vi "test-kalman-filter.vi"() -> (3 "ALL TESTS PASSED":bool)   [LabVIEW 2019]
uses:
  <vilib>/Rock Robotics/WPI/ThirdParty/JAS_Junk/TrajLib/LINEAR_SYSTEM.ctl
  <vilib>/Analysis/Matrix/Datatypes/RealMatrix.ctl
  <vilib>/Rock Robotics/WPI/ThirdParty/JAS_Junk/TrajLib/KALMAN_FILTER.ctl
  <vilib>/Rock Robotics/WPI/ThirdParty/JAS_Junk/TrajLib/Rotation_CreateAngle.vi
  <vilib>/Rock Robotics/WPI/ThirdParty/JAS_Junk/TrajLib/Translation_Create.vi
  <vilib>/Rock Robotics/WPI/ThirdParty/JAS_Junk/TrajLib/MatrixHelper_CoerceSize.vi
  <vilib>/Analysis/1siggen.llb/Gaussian White Noise.vi
  <vilib>/Analysis/Matrix/Numeric/Subtract/Subtract - RM,RM.vi
  <vilib>/Analysis/Matrix/Numeric/Add/Add - RM,RM.vi
  <vilib>/Rock Robotics/WPI/ThirdParty/JAS_Junk/TrajLib/Trajectory_Library.lvlib
  <vilib>/Analysis/Matrix/NI_Matrix.lvlib
panel:
  out "WhiteNoise":T1
  out "Error 3C":bool
  out "KalFilt Error 3B":bool
  out "KalFilt Error 3A":bool
  out "Test 1 Passed":bool
  out "max value 4B":dbl
  out "max value 4A":dbl
  out "Test 4 Passed":bool
  out "xHat 4":cluster{dbl[], dbl[]}(graph)
  out "Measurements 4":cluster{dbl[], dbl[]}(graph)
  out "Error 4A":bool
  out "Error 4B":bool
  out "KalFilt Error 4":bool
  out "KalFilt Test 4":T2
  out "max value 3B":dbl
  out "max value 3A":dbl
  out "Test 3 Passed":bool
  out "xHats 3":cluster{dbl[], dbl[]}(graph)
  out "Measurements 3":cluster{dbl[], dbl[]}(graph)
  out "Error 3A":bool
  out "Error 3B":bool
  out "KalFilt Error 3":bool
  out "KalFilt Test 3":T2
  out "Test 2 Passed":bool
  out "xHat 2":cluster{dbl[], dbl[]}(graph)
  out "Measurements 2":cluster{dbl[], dbl[]}(graph)
  out "Error 2B":bool
  out "Error 2A":bool
  out "KalFilt Error 2":bool
  out "KalFilt Test 2":T2
  out "KalFilt Error 1":bool
  out "KalFilt Test1":T2
  out "SwervObservError":bool
  out "SwervObservSystem":T3
  out "EllevError":bool
  out "ElevatorSystem":T3
  # "KALMAN FILTER"
  # "Steady State Gain  \n<States,Outputs>"
  # "State Estimate <Statess,1>"
  # "<States,States>"
  # "<States,Inputs>"
  # "<Outputs,States>"
  # "<Outputs,Inputs>"
  # "Steady State Gain  \n<States,Outputs>"
  # "State Estimate <Statess,1>"
  # "<States,States>"
  # "<States,Inputs>"
  # "<Outputs,States>"
  # "<Outputs,Inputs>"
  # "Steady State Gain  \n<States,Outputs>"
  # "State Estimate <Statess,1>"
  # "<States,States>"
  # "<States,Inputs>"
  # "<Outputs,States>"
  # "<Outputs,Inputs>"
  # "Steady State Gain  \n<States,Outputs>"
  # "State Estimate <Statess,1>"
  # "<States,States>"
  # "<States,Inputs>"
  # "<Outputs,States>"
  # "<Outputs,Inputs>"
  # "<States,States>"
  # "<States,Inputs>"
  # "<Outputs,States>"
  # "<Outputs,Inputs>"
  # "<States,States>"
  # "<States,Inputs>"
  # "<Outputs,States>"
  # "<Outputs,Inputs>"
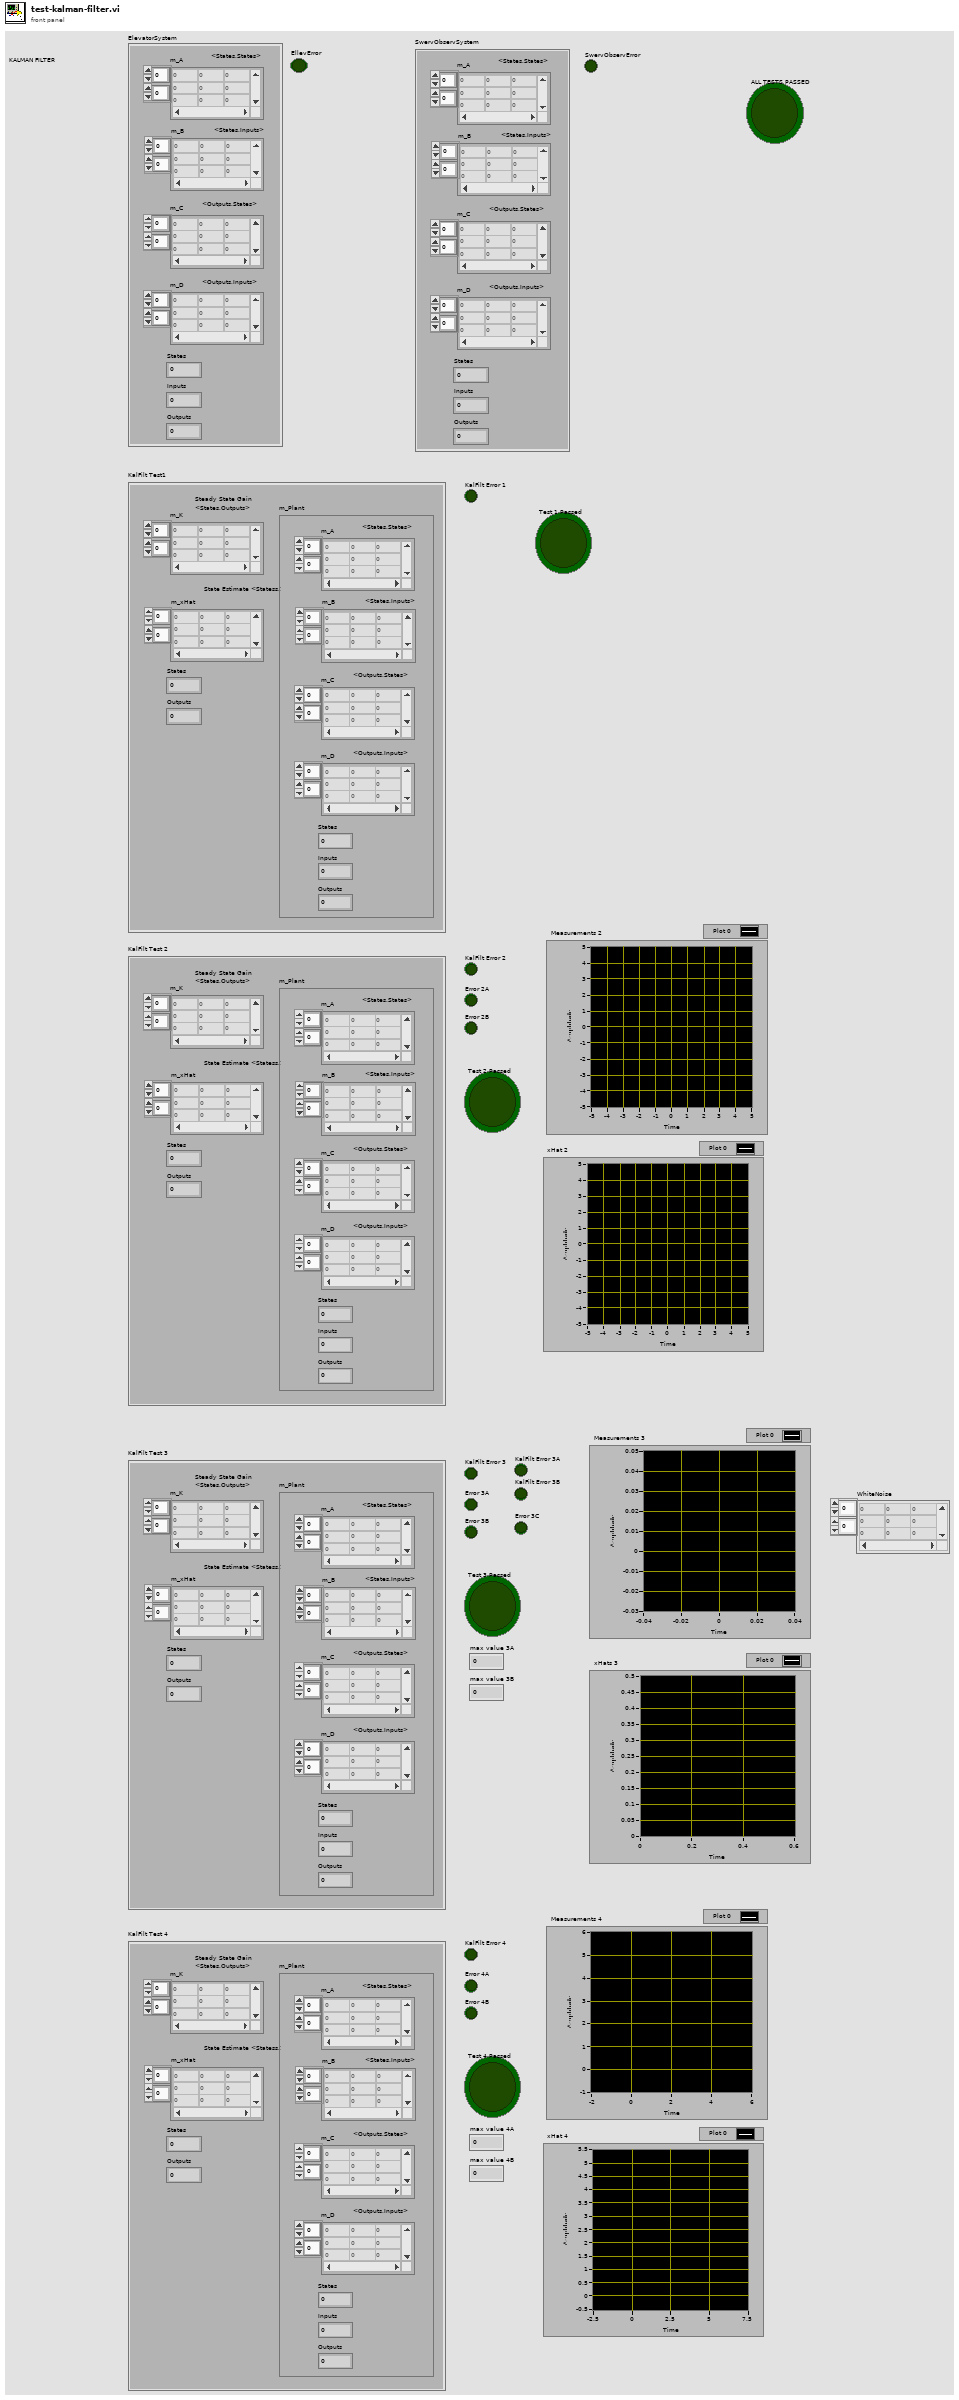
[diagram p1: front panel]
types:
  T1 = typedef "NI_Matrix.lvlib/RealMatrix.ctl" = dbl[][]
  T2 = typedef "Trajectory_Library.lvlib/KALMAN_FILTER.ctl" = cluster{"m_K":T1, "m_xHat":T1, "States":i32, "Outputs":i32, "m_Plant":T3}
  T3 = typedef "Trajectory_Library.lvlib/LINEAR_SYSTEM.ctl" = cluster{"m_A":T1, "m_B":T1, "m_C":T1, "m_D":T1, "States":i32, "Inputs":i32, "Outputs":i32}
  T4 = typedef "Trajectory_Library.lvlib/TRAJ_CONFIG.ctl" = cluster{"MaxVelocity":dbl, "Max Acceleration":dbl, "StartVelocity":dbl, "End Velocity":dbl, "Reversed":bool, "DiffDrKineConstntDefined":bool, "CentAcellConstntDefined":bool, "DiffDrVoltConstntDefined":bool, "DIFF_DRIVE_KINE_CONSTRAINT":T5, "CENTRIPETAL_ACCEL_CONSTRAINT":T7, "SwerveDrKineConstntDefined":bool, "SWERVE_DRIVE_KINE_CONSTRAINT":T8, "DIFF_DRIVE_VOLTAGE_CONSTRAINT":T11, "MECANUM_DRIVE_KINE_CONSTRAINT":T13, "MecanumDrKineConstntDefined":bool}
  T5 = typedef "Trajectory_Library.lvlib/TRAJ_CONSTRAINT_DIIF_DRIVE_KINEMATICS.ctl" = cluster{"Max Speed (M/S)":dbl, "DIFF_DRIVE_KINEMATICS":T6}
  T6 = typedef "Trajectory_Library.lvlib/DIFF_DRIVE_KINEMATICS.ctl" = cluster{"TrackWidth_Meters":dbl}
  T7 = typedef "Trajectory_Library.lvlib/TRAJ_CONSTRAINT_CENTRIPETAL_ACCEL.ctl" = cluster{"Max Cent Accel":dbl}
  T8 = typedef "Trajectory_Library.lvlib/TRAJ_CONSTRAINT_SWERVE_DRIVE_KINEMATICS.ctl" = cluster{"Max Speed (M/S)":dbl, "SwerveKinematics":T9}
  T9 = typedef "Trajectory_Library.lvlib/SWERVE_DRIVE_KINEMATICS.ctl" = cluster{"NumModules":i32, "InverseKinematics":T1, "ForwardKinematics":T1, "Modules":T10[], "PrevCoR":T10}
  T10 = typedef "Trajectory_Library.lvlib/TRANSLATION2D.ctl" = cluster{"X":dbl, "Y":dbl}
  T11 = typedef "Trajectory_Library.lvlib/TRAJ_CONSTRAINT_DIIF_DRIVE_VOLTAGE.ctl" = cluster{"Max Voltage":dbl, "DIFF_DRIVE_KINEMATICS":T6, "SIMPLE_MOTOR_FF":T12}
  T12 = typedef "Trajectory_Library.lvlib/SIMPLE_MOTOR_FF.ctl" = cluster{"Ks":dbl, "Kv":dbl, "Ka":dbl}
  T13 = typedef "Trajectory_Library.lvlib/TRAJ_CONSTRAINT_MECA_DRIVE_KINEMATICS.ctl" = cluster{"Max Speed (M/S)":dbl, "MECA_DRIVE_KINEMATICS":T14}
  T14 = typedef "Trajectory_Library.lvlib/MECA_DRIVE_KINEMATICS.ctl" = cluster{"FrontLeft":T10, "FrontRight":T10, "RearLeft":T10, "RearRight":T10, "InverseKinematics":T1, "ForwardKinematics":T1, "PrevCoR":T10}
  T15 = typedef "Trajectory_Library.lvlib/POSE2D.ctl" = cluster{"TRANSLATION":T10, "ROTATION":T16}
  T16 = typedef "Trajectory_Library.lvlib/ROTATION2D.ctl" = cluster{"VALUE":dbl, "COS":dbl, "SIN":dbl}
  T17 = typedef "Trajectory_Library.lvlib/TRAJECTORY.ctl" = cluster{"TotalTImeSecs":dbl, "States":T18[]}
  T18 = typedef "Trajectory_Library.lvlib/TRAJ_STATE.ctl" = cluster{"TimeSeconds":dbl, "Velocity":dbl, "Acceleration":dbl, "POSE":T15, "Curvature":dbl}
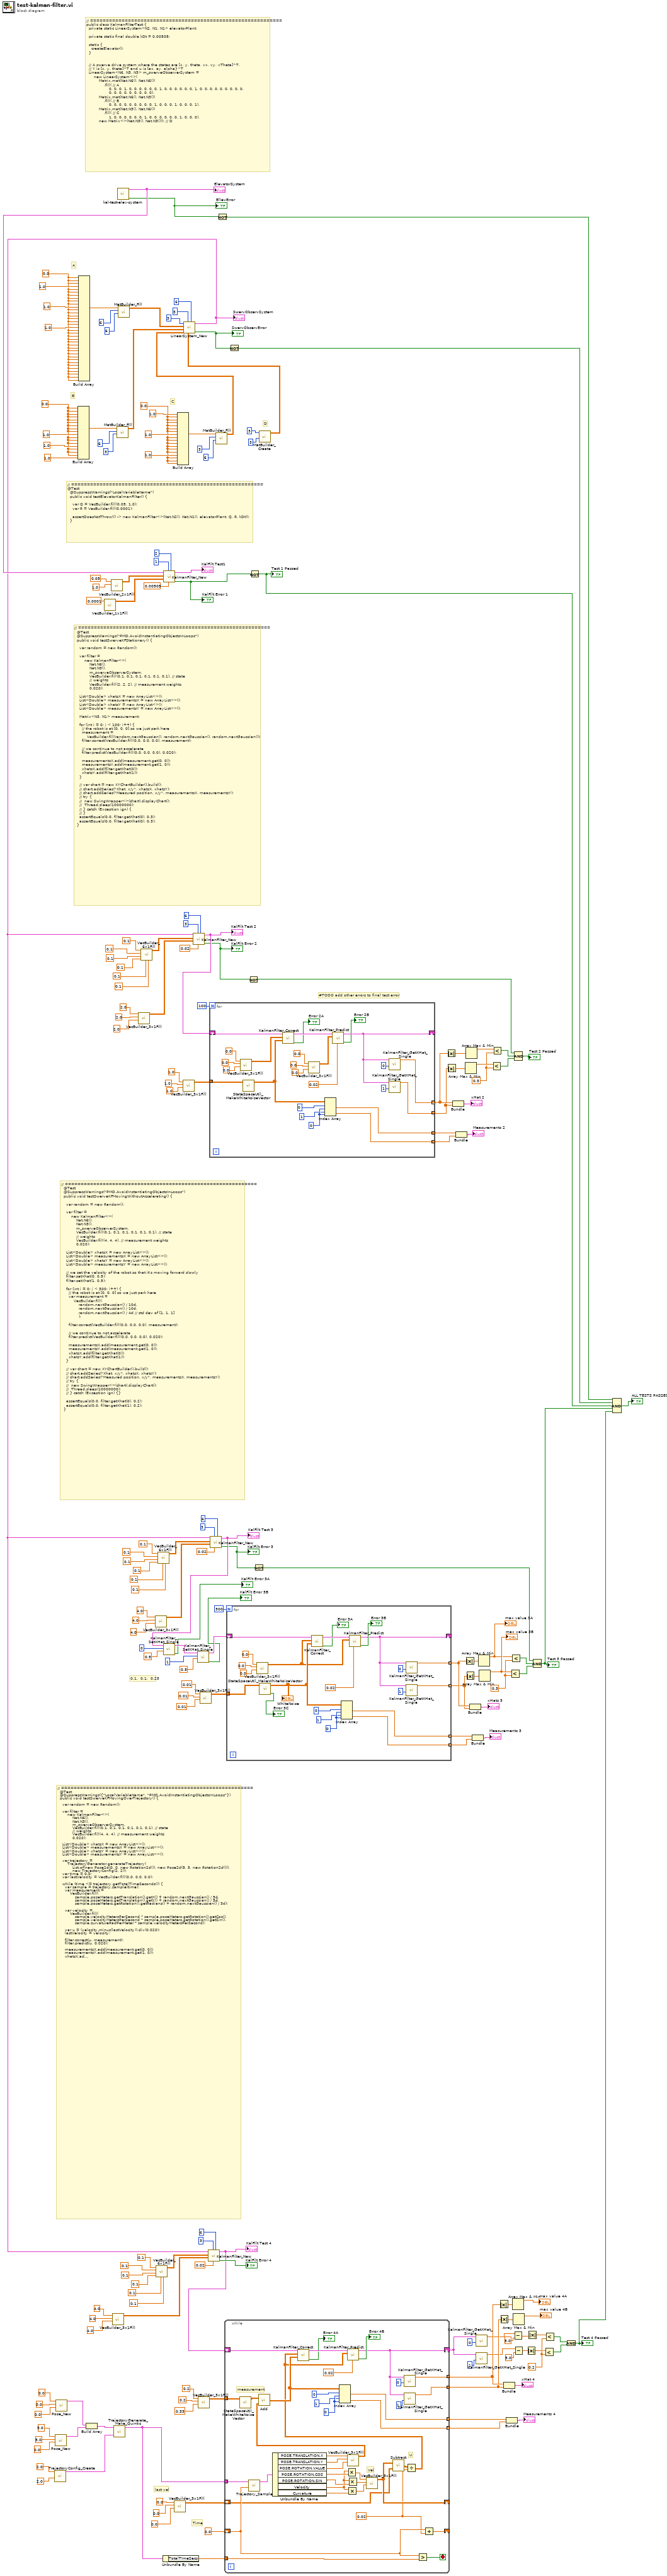
[diagram p0: block diagram]
diagram:
  w50 = 0.2 ("y")
  w89 = 0.3 ("y")
  w122 = 0.3 ("y")
  w169 = 0.0 ("element")
  w176 = 0.0 ("element")
  w184 = 0.0 ("element")
  # "0.1,  0.1,  0.25"
  # "#TODO add other errors to final test error"
  # "last vel"
  # "Time"
  # "// =============================================================\n  @Test\n  @SuppressWarnings(\"PMD.AvoidInstantiatingObjectsInLoops\")\n  public void testSwerveKFMovingWithoutAccelerating() {\n\n    var random = new Random();\n\n    var filter =\n        new KalmanFilter<>(\n            Nat.N6(),\n            Nat.N3(),\n            m_swerveObserverSystem,\n            VecBuilder.fill(0.1, 0.1, 0.1, 0.1, 0.1, 0.1), // state\n            // weights\n            VecBuilder.fill(4, 4, 4), // measurement weights\n            0.020);\n\n    List<Double> xhatsX = new ArrayList<>();\n    List<Double> measurementsX = new ArrayList<>();\n    List<Double> xhatsY = new ArrayList<>();\n    List<Double> measurementsY = new ArrayList<>();\n\n    // we set the velocity of the robot so that it's moving forward slowly\n    filter.setXhat(0, 0.5);\n    filter.setXhat(1, 0.5);\n\n    for (int i = 0; i < 300; i++) {\n      // the robot is at [0, 0, 0] so we just park here\n      var measurement =\n          VecBuilder.fill(\n              random.nextGaussian() / 10d,\n              random.nextGaussian() / 10d,\n              random.nextGaussian() / 4d // std dev of [1, 1, 1]\n              );\n\n      filter.correct(VecBuilder.fill(0.0, 0.0, 0.0), measurement);\n\n      // we continue to not accelerate\n      filter.predict(VecBuilder.fill(0.0, 0.0, 0.0), 0.020);\n\n      measurementsX.add(measurement.get(0, 0));\n      measurementsY.add(measurement.get(1, 0));\n      xhatsX.add(filter.getXhat(0));\n      xhatsY.add(filter.getXhat(1));\n    }\n\n    // var chart = new XYChartBuilder().build();\n    // chart.addSeries(\"Xhat, x/y\", xhatsX, xhatsY);\n    // chart.addSeries(\"Measured position, x/y\", measurementsX, measurementsY);\n    // try {\n    //  new SwingWrapper<>(chart).displayChart();\n    //  Thread.sleep(10000000);\n    // } catch (Exception ign) {}\n\n    assertEquals(0.0, filter.getXhat(0), 0.2);\n    assertEquals(0.0, filter.getXhat(1), 0.2);\n  }"
  # "// =============================================================\n  @Test\n  @SuppressWarnings(\"PMD.AvoidInstantiatingObjectsInLoops\")\n  public void testSwerveKFStationary() {\n\n    var random = new Random();\n\n    var filter =\n        new KalmanFilter<>(\n            Nat.N6(),\n            Nat.N3(),\n            m_swerveObserverSystem,\n            VecBuilder.fill(0.1, 0.1, 0.1, 0.1, 0.1, 0.1), // state\n            // weights\n            VecBuilder.fill(2, 2, 2), // measurement weights\n            0.020);\n\n    List<Double> xhatsX = new ArrayList<>();\n    List<Double> measurementsX = new ArrayList<>();\n    List<Double> xhatsY = new ArrayList<>();\n    List<Double> measurementsY = new ArrayList<>();\n\n    Matrix<N3, N1> measurement;\n\n    for (int i = 0; i < 100; i++) {\n      // the robot is at [0, 0, 0] so we just park here\n      measurement =\n          VecBuilder.fill(random.nextGaussian(), random.nextGaussian(), random.nextGaussian());\n      filter.correct(VecBuilder.fill(0.0, 0.0, 0.0), measurement);\n\n      // we continue to not accelerate\n      filter.predict(VecBuilder.fill(0.0, 0.0, 0.0), 0.020);\n\n      measurementsX.add(measurement.get(0, 0));\n      measurementsY.add(measurement.get(1, 0));\n      xhatsX.add(filter.getXhat(0));\n      xhatsY.add(filter.getXhat(1));\n    }\n\n    // var chart = new XYChartBuilder().build();\n    // chart.addSeries(\"Xhat, x/y\", xhatsX, xhatsY);\n    // chart.addSeries(\"Measured position, x/y\", measurementsX, measurementsY);\n    // try {\n    //  new SwingWrapper<>(chart).displayChart();\n    //  Thread.sleep(10000000);\n    // } catch (Exception ign) {\n    // }\n    assertEquals(0.0, filter.getXhat(0), 0.3);\n    assertEquals(0.0, filter.getXhat(0), 0.3);\n  }"
  # "// =============================================================\n@Test\n  @SuppressWarnings(\"LocalVariableName\")\n  public void testElevatorKalmanFilter() {\n\n    var Q = VecBuilder.fill(0.05, 1.0);\n    var R = VecBuilder.fill(0.0001);\n\n    assertDoesNotThrow(() -> new KalmanFilter<>(Nat.N2(), Nat.N1(), elevatorPlant, Q, R, kDt));\n  }"
  # "D"
  # "C"
  # "B"
  # "A"
  # "// =============================================================\npublic class KalmanFilterTest {\n  private static LinearSystem<N2, N1, N1> elevatorPlant;\n\n  private static final double kDt = 0.00505;\n\n  static {\n    createElevator();\n  }\n\n\n  // A swerve drive system where the states are [x, y, theta, vx, vy, vTheta]^T,\n  // Y is [x, y, theta]^T and u is [ax, ay, alpha}^T\n  LinearSystem<N6, N3, N3> m_swerveObserverSystem =\n      new LinearSystem<>(\n          Matrix.mat(Nat.N6(), Nat.N6())\n              .fill( // A\n                  0, 0, 0, 1, 0, 0, 0, 0, 0, 0, 1, 0, 0, 0, 0, 0, 0, 1, 0, 0, 0, 0, 0, 0, 0, 0, 0,\n                  0, 0, 0, 0, 0, 0, 0, 0, 0),\n          Matrix.mat(Nat.N6(), Nat.N3())\n              .fill( // B\n                  0, 0, 0, 0, 0, 0, 0, 0, 0, 1, 0, 0, 0, 1, 0, 0, 0, 1),\n          Matrix.mat(Nat.N3(), Nat.N6())\n              .fill( // C\n                  1, 0, 0, 0, 0, 0, 0, 1, 0, 0, 0, 0, 0, 0, 1, 0, 0, 0),\n          new Matrix<>(Nat.N3(), Nat.N3())); // D"
  # "// =============================================================\n  @Test\n  @SuppressWarnings({\"LocalVariableName\", \"PMD.AvoidInstantiatingObjectsInLoops\"})\n  public void testSwerveKFMovingOverTrajectory() {\n\n    var random = new Random();\n\n    var filter =\n        new KalmanFilter<>(\n            Nat.N6(),\n            Nat.N3(),\n            m_swerveObserverSystem,\n            VecBuilder.fill(0.1, 0.1, 0.1, 0.1, 0.1, 0.1), // state\n            // weights\n            VecBuilder.fill(4, 4, 4), // measurement weights\n            0.020);\n\n    List<Double> xhatsX = new ArrayList<>();\n    List<Double> measurementsX = new ArrayList<>();\n    List<Double> xhatsY = new ArrayList<>();\n    List<Double> measurementsY = new ArrayList<>();\n\n    var trajectory =\n        TrajectoryGenerator.generateTrajectory(\n            List.of(new Pose2d(0, 0, new Rotation2d()), new Pose2d(5, 5, new Rotation2d())),\n            new TrajectoryConfig(2, 2));\n    var time = 0.0;\n    var lastVelocity = VecBuilder.fill(0.0, 0.0, 0.0);\n\n    while (time <= trajectory.getTotalTimeSeconds()) {\n      var sample = trajectory.sample(time);\n      var measurement =\n          VecBuilder.fill(\n              sample.poseMeters.getTranslation().getX() + random.nextGaussian() / 5d,\n              sample.poseMeters.getTranslation().getY() + random.nextGaussian() / 5d,\n              sample.poseMeters.getRotation().getRadians() + random.nextGaussian() / 3d);\n\n      var velocity =\n          VecBuilder.fill(\n              sample.velocityMetersPerSecond * sample.poseMeters.getRotation().getCos(),\n              sample.velocityMetersPerSecond * sample.poseMeters.getRotation().getSin(),\n              sample.curvatureRadPerMeter * sample.velocityMetersPerSecond);\n\n      var u = (velocity.minus(lastVelocity)).div(0.020);\n      lastVelocity = velocity;\n\n      filter.correct(u, measurement);\n      filter.predict(u, 0.020);\n\n      measurementsX.add(measurement.get(0, 0));\n      measurementsY.add(measurement.get(1, 0));\n      xhatsX.add(filter.getXhat(0));\n      xhatsY.add(filter.getXhat(1));\n\n      time += 0.020;\n    }\n\n    // var chart = new XYChartBuilder().build();\n    // chart.addSeries(\"Xhat, x/y\", xhatsX, xhatsY);\n    // chart.addSeries(\"Measured position, x/y\", measurementsX, measurementsY);\n    // try {\n    //        new SwingWrapper<>(chart).displayChart();\n    //        Thread.sleep(10000000);\n    // } catch (Exception ign) {\n    // }\n\n    assertEquals(\n        trajectory.sample(trajectory.getTotalTimeSeconds()).poseMeters.getTranslation().getX(),\n        filter.getXhat(0),\n        0.2);\n    assertEquals(\n        trajectory.sample(trajectory.getTotalTimeSeconds()).poseMeters.getTranslation().getY(),\n        filter.getXhat(1),\n        0.2);\n  }\n}"
  n1 = call <vilib>:"TrajectoryConfig_Create.vi"("MaxAcceleration"=2.0, "MaxVelocity"=2.0) -> ("TRAJECTORY_CONFIG"=w35:T4)  [unwired: 9 in]
  n2 = call <vilib>:"Pose_New.vi"("Heading"=0.0, "Y"=5.0, "X"=5.0) -> ("out POSe"=w39:T15)  [unwired: 8 in]
  n3 = call <vilib>:"Pose_New.vi"("Heading"=0.0, "Y"=0.0, "X"=0.0) -> ("out POSe"=w40:T15)  [unwired: 8 in]
  n4 = Build Array(w176, w176, w176, w176, w176, w176, w176, w176, w176, 1.0 ("element"), w176, w176, w176, 1.0 ("element"), w176, w176, w176, 1.0 ("element")) -> (w181:dbl[])
  n5 = Build Array(w184, w184, w184, 1.0 ("element"), w184, w184, w184, w184, w184, w184, 1.0 ("element"), w184, w184, w184, w184, w184, w184, 1.0 ("element"), w184, w184, w184, w184, w184, w184, w184, w184, w184, w184, w184, w184, w184, w184, w184, w184, w184, w184) -> (w192:dbl[])
  n6 = Build Array(w40, w39) -> (w38:T15[])
  n7 = call <vilib>:"VecBuilder_1x1Fill.vi"("R0_C0"=0.0001) -> ("output matrix"=w155:T1)  [unwired: 10 in]
  n8 = call <vilib>:"VecBuilder_2x1Fill.vi"("R1"=1.0, "R0"=0.05) -> ("output matrix"=w156:T1)  [unwired: 9 in]
  n9 = call <vilib>:"VecBuilder_3x1Fill.vi"("R2"=4.0, "R1"=4.0, "R0"=4.0 ("R0_C0")) -> ("output matrix"=w73:T1)  [unwired: 8 in]
  n10 = call <vilib>:"TrajectoryGenerate_Make_Quintic.vi"("traj_config"=w35, "waypointPOSE"=w38) -> ("TRAJECTORY"=w32:T17)  [unwired: 8 in, 1 out]
  n11 = call <vilib>:"MatBuilder_Fill.vi"("Columns"=3, "Rows"=6, "Value List"=w181) -> ("output matrix"=w166:T1)  [unwired: 8 in]
  n12 = call "kal-test-elev-system.vi"() -> ("Error"=w13:bool, "ElevatorSystem"=w162:T3)  [unwired: 10 in]
  "ElevatorSystem" <- w162
  "EllevError" <- w13
  n13 = call <vilib>:"MatBuilder_Fill.vi"("Columns"=6, "Rows"=6, "Value List"=w192) -> ("output matrix"=w182:T1)  [unwired: 8 in]
  n14 = call <vilib>:"VecBuilder_3x1Fill.vi"("R2"=2.0, "R1"=2.0, "R0"=2.0 ("R0_C0")) -> ("output matrix"=w146:T1)  [unwired: 8 in]
  n15 = call <vilib>:"VecBuilder_6x1Fill.vi"("R5"=0.1, "R4"=0.1, "R3"=0.1, "R2"=0.1, "R1"=0.1, "R0"=0.1) -> ("output matrix"=w147:T1)  [unwired: 5 in]
  n16 = call <vilib>:"VecBuilder_3x1Fill.vi"("R2"=4.0, "R1"=4.0, "R0"=4.0 ("R0_C0")) -> ("output matrix"=w112:T1)  [unwired: 8 in]
  n17 = call <vilib>:"VecBuilder_6x1Fill.vi"("R5"=0.1, "R4"=0.1, "R3"=0.1, "R2"=0.1, "R1"=0.1, "R0"=0.1) -> ("output matrix"=w74:T1)  [unwired: 5 in]
  n18 = call <vilib>:"VecBuilder_6x1Fill.vi"("R5"=0.1, "R4"=0.1, "R3"=0.1, "R2"=0.1, "R1"=0.1, "R0"=0.1) -> ("output matrix"=w113:T1)  [unwired: 5 in]
  n19 = Unbundle By Name(w32) -> ("TotalTImeSecs"=w31:dbl)
  n20 = call <vilib>:"KalmanFilter_New.vi"("States"=2, "dt_Seconds"=0.00505, "Outputs"=1, "MeasurementStdDevs"=w155, "StateStdDevs"=w156, "Plant"=w162) -> ("Error"=w15:bool, "KalmanFilter"=→"KalFilt Test1":T2)  [unwired: 4 in]
  "KalFilt Error 1" <- w15
  n21 = call <vilib>:"VecBuilder_3x1Fill.vi"("R2"=0.0, "R1"=0.0, "R0"=0.0) -> ("output matrix"=w27:T1)  [unwired: 8 in]
  n22 = Build Array(1.0 ("element"), w169, w169, w169, w169, w169, w169, 1.0 ("element"), w169, w169, w169, w169, w169, w169, 1.0 ("element"), w169, w169, w169) -> (w175:dbl[])
  n23 = call <vilib>:"VecBuilder_3x1Fill.vi"("R2"=1.0, "R1"=1.0, "R0"=1.0) -> ("output matrix"=w134:T1)  [unwired: 8 in]
  n24 = call <vilib>:"VecBuilder_3x1Fill.vi"("R2"=0.33, "R1"=0.2, "R0"=0.2) -> ("output matrix"=w61:T1)  [unwired: 8 in]
  n25 = call <vilib>:"VecBuilder_3x1Fill.vi"("R2"=0.01, "R1"=0.01, "R0"=0.01) -> ("output matrix"=w100:T1)  [unwired: 8 in]
  n26 = call <vilib>:"MatBuilder_Fill.vi"("Columns"=6, "Rows"=3, "Value List"=w175) -> ("output matrix"=w165:T1)  [unwired: 8 in]
  n27 = Not(x=w13) -> (.not. x?=w12:bool)
  n28 = Not(x=w15) -> (.not. x?=w9:bool)
  "Test 1 Passed" <- w9
  n29 = call <vilib>:"MatBuilder_Create.vi"("Columns"=3, "Rows"=3) -> ("output matrix"=w164:T1)  [unwired: 9 in]
  n30 = call <vilib>:"LinearSystem_New.vi"("States"=6, "D"=w164, "Inputs"=3, "C"=w165, "B"=w166, "A"=w182, "Outputs"=3) -> ("Size Coerced"=w11:bool, "Linearsystem"=w47:T3)  [unwired: 3 in]
  "SwervObservSystem" <- w47
  "SwervObservError" <- w11
  n31 = call <vilib>:"KalmanFilter_New.vi"("States"=6, "dt_Seconds"=0.02, "Outputs"=3, "MeasurementStdDevs"=w146, "StateStdDevs"=w147, "Plant"=w47) -> ("Error"=w8:bool, "KalmanFilter"=w133:T2)  [unwired: 4 in]
  "KalFilt Test 2" <- w133
  "KalFilt Error 2" <- w8
  n32 = call <vilib>:"KalmanFilter_New.vi"("States"=6, "dt_Seconds"=0.02, "Outputs"=3, "MeasurementStdDevs"=w73, "StateStdDevs"=w74, "Plant"=w47) -> ("Error"=→"KalFilt Error 4":bool, "KalmanFilter"=w33:T2)  [unwired: 4 in]
  "KalFilt Test 4" <- w33
  n33 = for {
    N: 100 -> [_]
    tunnel: w134 -> [w217]
    shift-right: [w195] -> _
    shift-left: w133 -> [w213]
    tunnel: [w199] -> w131 mode=indexing
    tunnel: [w198] -> w130 mode=indexing
    tunnel: [w193] -> w128 mode=indexing
    tunnel: [w194] -> w127 mode=indexing
    w202 = 0 ("index (col)")
    n34 = call <vilib>:"VecBuilder_3x1Fill.vi"("R2"=0.0, "R1"=0.0, "R0"=0.0) -> ("output matrix"=w212:T1)  [unwired: 8 in]
    n35 = call <vilib>:"StateSpaceUtil_MakeWhiteNoiseVector.vi"("StdDevs"=w217) -> ("WhiteNoise"=w203:T1)  [unwired: 9 in, 1 out]
    n36 = call <vilib>:"KalmanFilter_Correct.vi"("Y"=w203, "U"=w212, "in KalmanFilter"=w213) -> ("Error"=→"Error 2A":bool, "out KalmanFilter"=w208:T2)  [unwired: 7 in]
    n37 = call <vilib>:"VecBuilder_3x1Fill.vi"("R2"=0.0, "R1"=0.0, "R0"=0.0) -> ("output matrix"=w207:T1)  [unwired: 8 in]
    n38 = Index Array(array=w203, index (row) #1=0 ("index (row)"), index (col) #1=w202, index (row) #2=1 ("index (row)"), index (col) #2=w202) -> (element #1=w199:dbl, element #2=w198:dbl)
    n39 = call <vilib>:"KalmanFilter_Predict.vi"("dT_Seconds"=0.02, "U"=w207, "in KalmanFilter"=w208) -> ("Error"=→"Error 2B":bool, "out KalmanFilter"=w195:T2)  [unwired: 7 in]
    n40 = call <vilib>:"KalmanFilter_GetXHat_Single.vi"("Row"=0, "in KalmanFilter"=w195) -> ("xHat"=w193:dbl)  [unwired: 9 in]
    n41 = call <vilib>:"KalmanFilter_GetXHat_Single.vi"("Row"=1, "in KalmanFilter"=w195) -> ("xHat"=w194:dbl)  [unwired: 9 in]
  }
  n42 = call <vilib>:"KalmanFilter_New.vi"("States"=6, "dt_Seconds"=0.02, "Outputs"=3, "MeasurementStdDevs"=w112, "StateStdDevs"=w113, "Plant"=w47) -> ("Error"=w6:bool, "KalmanFilter"=w86:T2)  [unwired: 4 in]
  "KalFilt Test 3" <- w86
  "KalFilt Error 3" <- w6
  n43 = call <vilib>:"KalmanFilter_SetXHat_Single.vi"("xHat"=0.5, "Row"=0, "in KalmanFilter"=w86) -> ("Error"=→"KalFilt Error 3A":bool, "out KalmanFilter"=w85:T2)  [unwired: 7 in]
  n44 = call <vilib>:"KalmanFilter_SetXHat_Single.vi"("xHat"=0.5, "Row"=1, "in KalmanFilter"=w85) -> ("Error"=→"KalFilt Error 3B":bool, "out KalmanFilter"=w84:T2)  [unwired: 7 in]
  n45 = while {
    tunnel: w61 -> [w257]
    shift-right: [w244] -> w24
    shift-left: w33 -> [w256]
    tunnel: [w248] -> w59 mode=indexing
    tunnel: [w247] -> w58 mode=indexing
    tunnel: [w242] -> w56 mode=indexing
    tunnel: [w243] -> w55 mode=indexing
    shift-right: [w240] -> _
    shift-left: 0.0 -> [w223]
    tunnel: w32 -> [w241]
    tunnel: w31 -> [w238]
    shift-right: [w222] -> _
    shift-left: w27 -> [w221]
    stop <- w239 stop-if-true
    w219 = 0.02 ("y")
    w251 = 0 ("index (col)")
    # "U"
    # "Vel"
    # "measurement"
    n46 = call <vilib>:"StateSpaceUtil_MakeWhiteNoiseVector.vi"("StdDevs"=w257) -> ("WhiteNoise"=w233:T1)  [unwired: 9 in, 1 out]
    n47 = call <vilib>:"Trajectory_Sample.vi"("Time"=w223, "InputTRAJECTORY"=w241) -> ("OutputTRAJ_STATE"=w237:T18)  [unwired: 9 in]
    n48 = Unbundle By Name(w237) -> ("POSE.TRANSLATION.X"=w236:dbl, "POSE.TRANSLATION.Y"=w235:dbl, "POSE.ROTATION.VALUE"=w234:dbl, "POSE.ROTATION.COS"=w230:dbl, "POSE.ROTATION.SIN"=w229:dbl, "Velocity"=w228:dbl, "Curvature"=w227:dbl)
    n49 = Multiply(x=w228, y=w230) -> (x*y=w226:dbl)
    n50 = Multiply(x=w228, y=w227) -> (x*y=w224:dbl)
    n51 = Multiply(x=w228, y=w229) -> (x*y=w225:dbl)
    n52 = call <vilib>:"VecBuilder_3x1Fill.vi"("R2"=w234, "R1"=w235, "R0"=w236) -> ("output matrix"=w232:T1)  [unwired: 8 in]
    n53 = call-poly <vilib>:"Add.vi"("Real Matrix B"=w232, "Real Matrix A"=w233) -> ("A + B"=w231:T1)
    n54 = Index Array(array=w231, index (row) #1=0 ("index (row)"), index (col) #1=w251, index (row) #2=1 ("index (row)"), index (col) #2=w251) -> (element #1=w248:dbl, element #2=w247:dbl)
    n55 = call <vilib>:"VecBuilder_3x1Fill.vi"("R2"=w224, "R1"=w225, "R0"=w226) -> ("output matrix"=w222:T1)  [unwired: 8 in]
    n56 = call-poly <vilib>:"Subtract.vi"("Real Matrix B"=w221, "Real Matrix A"=w222) -> ("A - B"=w220:T1)
    n57 = Divide(x=w220, y=w219) -> (x/y=w218:T1)
    n58 = call <vilib>:"KalmanFilter_Correct.vi"("Y"=w231, "U"=w218, "in KalmanFilter"=w256) -> ("Error"=→"Error 4A":bool, "out KalmanFilter"=w255:T2)  [unwired: 7 in]
    n59 = call <vilib>:"KalmanFilter_Predict.vi"("dT_Seconds"=0.02, "U"=w218, "in KalmanFilter"=w255) -> ("Error"=→"Error 4B":bool, "out KalmanFilter"=w244:T2)  [unwired: 7 in]
    n60 = call <vilib>:"KalmanFilter_GetXHat_Single.vi"("Row"=0, "in KalmanFilter"=w244) -> ("xHat"=w242:dbl)  [unwired: 9 in]
    n61 = call <vilib>:"KalmanFilter_GetXHat_Single.vi"("Row"=1, "in KalmanFilter"=w244) -> ("xHat"=w243:dbl)  [unwired: 9 in]
    n62 = Greater?(x=w223, y=w238) -> (0:w239:bool)
    n63 = Add(x=w223, y=w219) -> (x+y=w240:dbl)
  }
  n64 = for {
    N: 300 -> [_]
    tunnel: w100 -> [w279]
    shift-right: [w262] -> _
    shift-left: w84 -> [w275]
    tunnel: [w266] -> w98 mode=indexing
    tunnel: [w265] -> w97 mode=indexing
    tunnel: [w260] -> w95 mode=indexing
    tunnel: [w261] -> w94 mode=indexing
    w269 = 0 ("index (col)")
    n65 = call <vilib>:"VecBuilder_3x1Fill.vi"("R2"=0.0, "R1"=0.0, "R0"=0.0) -> ("output matrix"=w259:T1)  [unwired: 8 in]
    n66 = call <vilib>:"StateSpaceUtil_MakeWhiteNoiseVector.vi"("StdDevs"=w279) -> ("Size Coerced"=→"Error 3C":bool, "WhiteNoise"=w270:T1)  [unwired: 9 in]
    "WhiteNoise" <- w270
    n67 = call <vilib>:"KalmanFilter_Correct.vi"("Y"=w270, "U"=w259, "in KalmanFilter"=w275) -> ("Error"=→"Error 3A":bool, "out KalmanFilter"=w274:T2)  [unwired: 7 in]
    n68 = Index Array(array=w270, index (row) #1=0 ("index (row)"), index (col) #1=w269, index (row) #2=1 ("index (row)"), index (col) #2=w269) -> (element #1=w266:dbl, element #2=w265:dbl)
    n69 = call <vilib>:"KalmanFilter_Predict.vi"("dT_Seconds"=0.02, "U"=w259, "in KalmanFilter"=w274) -> ("Error"=→"Error 3B":bool, "out KalmanFilter"=w262:T2)  [unwired: 7 in]
    n70 = call <vilib>:"KalmanFilter_GetXHat_Single.vi"("Row"=0, "in KalmanFilter"=w262) -> ("xHat"=w260:dbl)  [unwired: 9 in]
    n71 = call <vilib>:"KalmanFilter_GetXHat_Single.vi"("Row"=1, "in KalmanFilter"=w262) -> ("xHat"=w261:dbl)  [unwired: 9 in]
  }
  n72 = Not(x=w11) -> (.not. x?=w10:bool)
  n73 = Not(x=w8) -> (.not. x?=w7:bool)
  n74 = Not(x=w6) -> (.not. x?=w5:bool)
  n75 = Absolute Value(x=w128) -> (abs(x)=w125:dbl[])
  n76 = Absolute Value(x=w127) -> (abs(x)=w126:dbl[])
  n77 = Bundle(w128, w127) -> (→"xHat 2":cluster{dbl[], dbl[]})  [unwired: 1 in]
  n78 = Bundle(w131, w130) -> (→"Measurements 2":cluster{dbl[], dbl[]})  [unwired: 1 in]
  n79 = Absolute Value(x=w95) -> (abs(x)=w92:dbl[])
  n80 = Absolute Value(x=w94) -> (abs(x)=w93:dbl[])
  n81 = Array Max & Min(array=w126) -> (max value=w124:dbl)  [unwired: 3 out]
  n82 = Array Max & Min(array=w125) -> (max value=w123:dbl)  [unwired: 3 out]
  n83 = Bundle(w95, w94) -> (→"xHats 3":cluster{dbl[], dbl[]})  [unwired: 1 in]
  n84 = Bundle(w98, w97) -> (→"Measurements 3":cluster{dbl[], dbl[]})  [unwired: 1 in]
  n85 = call <vilib>:"KalmanFilter_GetXHat_Single.vi"("Row"=0, "in KalmanFilter"=w24) -> ("xHat"=w19:dbl)  [unwired: 9 in]
  n86 = call <vilib>:"KalmanFilter_GetXHat_Single.vi"("Row"=1, "in KalmanFilter"=w24) -> ("xHat"=w18:dbl)  [unwired: 9 in]
  n87 = Array Max & Min(array=w92) -> (max value=w90:dbl)  [unwired: 3 out]
  "max value 3A" <- w90
  n88 = Array Max & Min(array=w93) -> (max value=w91:dbl)  [unwired: 3 out]
  "max value 3B" <- w91
  n89 = Less?(x=w124, y=w122) -> (x < y?=w120:bool)
  n90 = Less?(x=w123, y=w122) -> (x < y?=w121:bool)
  n91 = Absolute Value(x=w56) -> (abs(x)=w53:dbl[])
  n92 = Absolute Value(x=w55) -> (abs(x)=w54:dbl[])
  n93 = Bundle(w56, w55) -> (→"xHat 4":cluster{dbl[], dbl[]})  [unwired: 1 in]
  n94 = Bundle(w59, w58) -> (→"Measurements 4":cluster{dbl[], dbl[]})  [unwired: 1 in]
  n95 = Less?(x=w91, y=w89) -> (x < y?=w87:bool)
  n96 = Less?(x=w90, y=w89) -> (x < y?=w88:bool)
  n97 = Array Max & Min(array=w53) -> (max value=→"max value 4A":dbl)  [unwired: 3 out]
  n98 = Subtract(x=w19, y=5.0) -> (x-y=w21:dbl)
  n99 = Array Max & Min(array=w54) -> (max value=→"max value 4B":dbl)  [unwired: 3 out]
  n100 = Subtract(x=w18, y=5.0) -> (x-y=w20:dbl)
  n101 = Compound Arithmetic op=AND(w7, w121, w120) -> (→"Test 2 Passed":bool)
  n102 = Absolute Value(x=w20) -> (abs(x)=w22:dbl)
  n103 = Absolute Value(x=w21) -> (abs(x)=w23:dbl)
  n104 = Compound Arithmetic op=AND(w5, w88, w87) -> (w4:bool)
  "Test 3 Passed" <- w4
  n105 = Less?(x=w22, y=w50) -> (x < y?=w48:bool)
  n106 = Less?(x=w23, y=w50) -> (x < y?=w49:bool)
  n107 = And(x=w49, y=w48) -> (x .and. y?=w3:bool)
  "Test 4 Passed" <- w3
  n108 = Compound Arithmetic op=AND(w12, w10, w9, w4, w3) -> (→"ALL TESTS PASSED":bool)
